vi "ReadInfoStatus.vi"() -> ()   [LabVIEW 2017]
doc: "This example demonstrates how to query an XML document by using an XPath expression and returns all the nodes that match the XPath expression."
uses:
  <vilib>/xml/Load XML File.vi
  <vilib>/xml/Close Reference(Node).vi
  <resource>/objmgr/DOMUserDefRef.rc
  <vilib>/xml/NI_XML.lvlib
panel:
  in  "stop":bool
  in  "error in (no error)":errorcluster
  out "error out":errorcluster
  in  "XPath Expression 2":string="/COOLER_STATUS/LIST_OF_PROPERTIES/PROPERTY"
  out "Status Results":string[](array[string])
  in  "path to XML document":path=path "C:/Users/User/AppData/Roaming/CryoConnector/811158/status.xml"
  in  "XPath Expression":string="/COOLER_STATUS/LIST_OF_INFO/INFO"
  out "Info Results":string[](array[string])
  # "Overview: Demonstrates the use of the XML Parser VIs and functions to search an XML string for multiple nodes (tags) that match a given XPath search expression.\nInstructions:\nRun the VI."
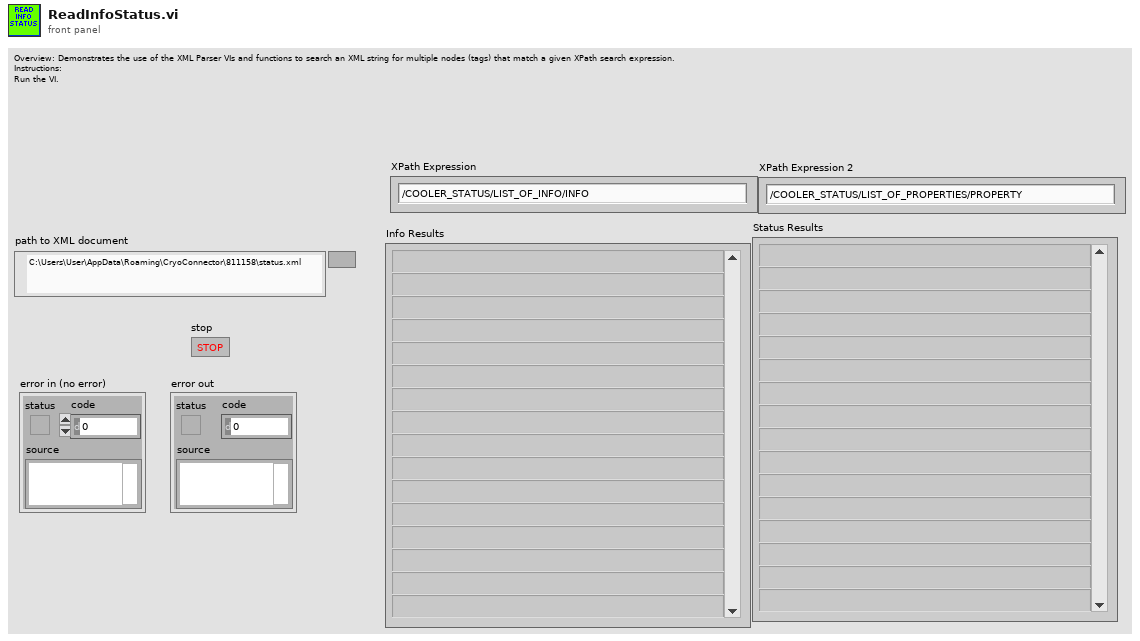
[diagram p1: front panel]
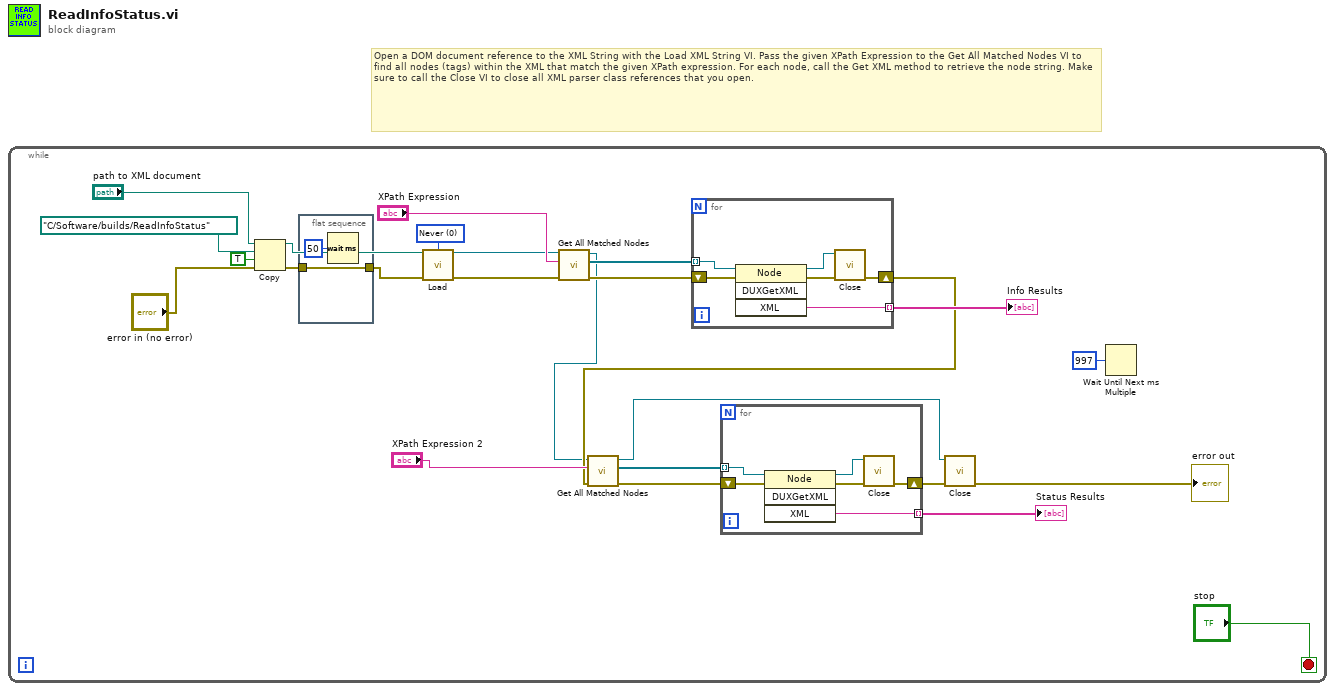
[diagram p0: block diagram]
diagram:
  # "Open a DOM document reference to the XML String with the Load XML String VI. Pass the given XPath Expression to the Get All Matched Nodes VI to find all nodes (tags) within the XML that match the given XPath expression. For each node, call the Get XML method to retrieve the node string. Make sure to call the Close VI to close all XML parser class references that you open."
  n1 = while {
    stop <- "stop" stop-if-true
    w9 = 0 items=["Never", "Always", "Auto"] ("validate on load (Auto)")
    n2 = Copy(8:"error in (no error)", 9:TRUE ("overwrite (F)"), 10:path "C:/Software/builds/ReadInfoStatus" ("target path (use dialog)"), 11:"path to XML document") -> (0:w3:errorcluster, 3:w6:path)  [unwired: 1 in, 1 out]
    n3 = flat-sequence {
      tunnel: w3 -> [w27]
      tunnel: [w27] -> w2
      frame #0 {
        n4 = Wait (ms)(milliseconds to wait=u32 50) -> ()  [unwired: 1 out]
      }
    }
    n5 = call-poly <vilib>:"Load.vi"("path to XML document"=w6, "validate on load (Auto)"=w9, "error in (no error)"=w2) -> ("DOM document out"=w15:refnum<k20>, "error out"=w21:errorcluster)  [unwired: 10 in, 1 out]
    n6 = call <vilib>:"Get All Matched Nodes.vi"("error in (no error)"=w21, "XPath expression"="XPath Expression", "node in"=w15) -> ("error out"=w24:errorcluster, "node result array"=w25:refnum<k20>[], "node out"=w12:refnum<k20>)  [unwired: 6 out]
    n7 = for {
      tunnel: w25 -> [w35] mode=indexing
      shift-right: [w37] -> w13
      shift-left: w24 -> [w36]
      tunnel: [w34] -> w22 mode=indexing
      n8 = invoke on="Invoke Node" class="Node" method="DUXGetXML"(reference=w35, error in=w36) -> (reference out=w38:refnum<k20>, error out=w39:errorcluster, "XML"=w34:string)  [unwired: 2 in, 1 out]
      n9 = call-poly <vilib>:"Close.vi"("error in (no error)"=w39, "node"=w38) -> ("error out"=w37:errorcluster)  [unwired: 7 out]
    }
    "Info Results" <- w22
    n10 = call <vilib>:"Get All Matched Nodes.vi"("error in (no error)"=w13, "XPath expression"="XPath Expression 2", "node in"=w12) -> ("error out"=w17:errorcluster, "node result array"=w16:refnum<k20>[], "node out"=w19:refnum<k20>)  [unwired: 6 out]
    n11 = for {
      tunnel: w16 -> [w29] mode=indexing
      shift-right: [w31] -> w18
      shift-left: w17 -> [w30]
      tunnel: [w28] -> w20 mode=indexing
      n12 = invoke on="Invoke Node" class="Node" method="DUXGetXML"(reference=w29, error in=w30) -> (reference out=w32:refnum<k20>, error out=w33:errorcluster, "XML"=w28:string)  [unwired: 2 in, 1 out]
      n13 = call-poly <vilib>:"Close.vi"("error in (no error)"=w33, "node"=w32) -> ("error out"=w31:errorcluster)  [unwired: 7 out]
    }
    "Status Results" <- w20
    n14 = call-poly <vilib>:"Close.vi"("error in (no error)"=w18, "node"=w19) -> ("error out"=→"error out":errorcluster)  [unwired: 7 out]
    n15 = Wait Until Next ms Multiple(millisecond multiple=u32 997) -> ()  [unwired: 1 out]
  }
